vi "History Points Holder.vi"(2 "Actions":T1=enum."Read", 7 "(x, y) Points":dbl[](array[numeric]), 13 "Zero Position (x, y)":dbl[](array[numeric])) -> (8 "History Points":cluster{i16[], i16[]})   [LabVIEW 2016]
uses:
  XY Sample Stage Controls/History Actions.ctl
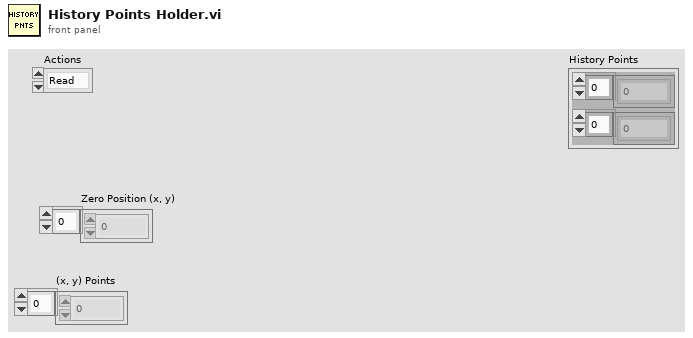
[diagram p1: front panel]
types:
  T1 = typedef "History Actions.ctl" = enum16{"Reset", "Write", "Read", "Set Zero"}
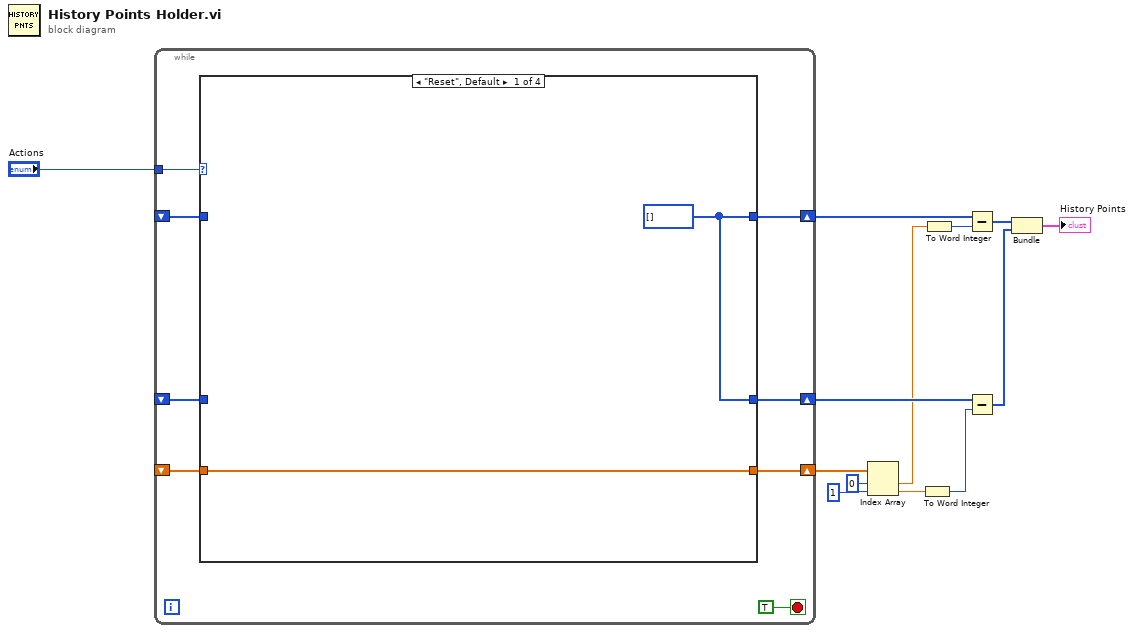
[diagram p0: block diagram]
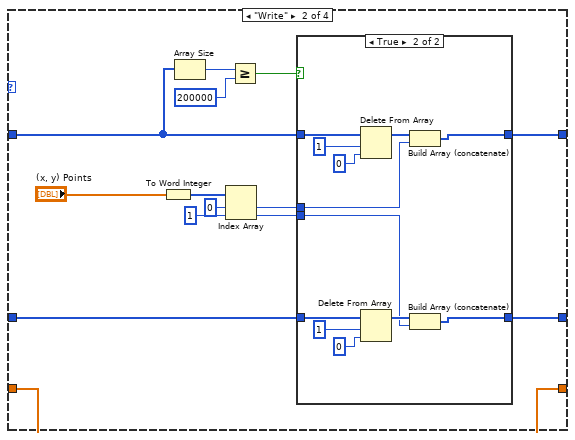
[diagram p2: hidden frame]
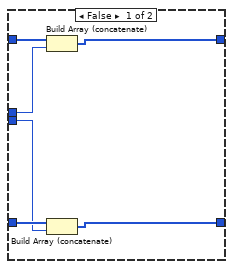
[diagram p3: hidden frame]
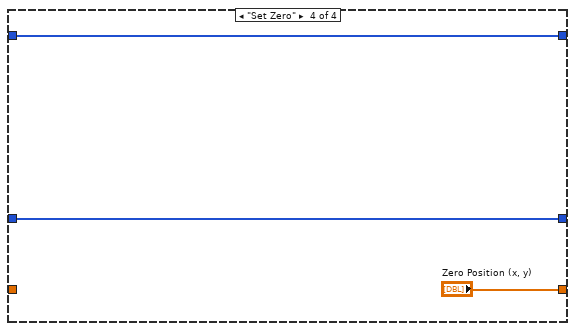
[diagram p5: hidden frame]
diagram:
  n1 = while {
    shift-right: [w19] -> w7
    shift-left: _ -> [w17]
    shift-right: [w18] -> w8
    shift-left: _ -> [w16]
    tunnel: "Actions" -> [w20]
    shift-right: [w15] -> w11
    shift-left: _ -> [w14]
    stop <- TRUE stop-if-true
    n2 = case shown="\"Reset\", Default" w20 {
      tunnel: [w23 w27 w58 w61] -> w19
      tunnel: [w23 w26 w57 w60] -> w18
      tunnel: w17 -> [_ w31 w58 w61]
      tunnel: w16 -> [_ w30 w57 w60]
      tunnel: [w22 w24 w56 "Zero Position (x, y)"] -> w15
      tunnel: w14 -> [w22 w24 w56 _]
      frame "Reset", Default {
        w23 = i16[] []
      }
      frame "Write" {
        n3 = To Word Integer(number="(x, y) Points") -> (16bit integer=w25:i16[])
        n4 = Array Size(array=w31) -> (size(s)=w37:i32)
        n5 = Index Array(array=w25, index #1=0 ("index"), index #2=1 ("index")) -> (element #1=w29:i16, element #2=w28:i16)
        n6 = Greater Or Equal?(x=w37, y=200000) -> (x >= y?=w35:bool)
        n7 = case shown="True" w35 {
          tunnel: w31 -> [w43 w55]
          tunnel: w30 -> [w42 w50]
          tunnel: w29 -> [w40 w47]
          tunnel: w28 -> [w41 w46]
          tunnel: [w39 w45] -> w27
          tunnel: [w38 w44] -> w26
          frame False {
            n8 = Build Array (concatenate)(w43, w40) -> (w39:i16[])
            n9 = Build Array (concatenate)(w42, w41) -> (w38:i16[])
          }
          frame True {
            n10 = Delete From Array(array=w55, length=1, index=0 ("length")) -> (array with subset deleted=w49:i16[])  [unwired: 1 out]
            n11 = Delete From Array(array=w50, length=1, index=0 ("length")) -> (array with subset deleted=w48:i16[])  [unwired: 1 out]
            n12 = Build Array (concatenate)(w49, w47) -> (w45:i16[])
            n13 = Build Array (concatenate)(w48, w46) -> (w44:i16[])
          }
        }
      }
      frame "Read" {
      }
      frame "Set Zero" {
      }
    }
  }
  n14 = Index Array(array=w11, index #1=0 ("index"), index #2=1 ("index")) -> (element #1=w3:dbl, element #2=w4:dbl)
  n15 = To Word Integer(number=w4) -> (16bit integer=w2:i16)
  n16 = To Word Integer(number=w3) -> (16bit integer=w1:i16)
  n17 = Subtract(x=w7, y=w1) -> (x-y=w6:i16[])
  n18 = Subtract(x=w8, y=w2) -> (x-y=w5:i16[])
  n19 = Bundle(w6, w5) -> (→"History Points":cluster{i16[], i16[]})  [unwired: 1 in]
